vi "stitchingModeOffset.vi"(8 "Offset":dbl, 9 "Data In":dbl[][][](array[numeric])) -> (2 "Stitched Data Out":dbl[][](array[numeric]))   [LabVIEW 2020, in "horiba.lvlib" / "CCD.lvclass"]
doc: "Stitches spectra based on simple cut-off modus."
uses:
  CCD.lvclass
  4c98e68f-fed8-44bd-a6f6-c5aabdf5d44d.vi
  <vilib>/Array/Sort 2D Array - Pop Stack.vi
  <vilib>/Array/Sort 2D Array - Push Stack.vi
  4c98e68f-fed8-44bd-a6f6-c5aabdf5d44d.vi/269d4b3b-47f5-49e3-8884-44851e4dd9d5.vi
  4c98e68f-fed8-44bd-a6f6-c5aabdf5d44d.vi/6d99389c-673d-4efb-bf33-19b32bcf4cf8.vi
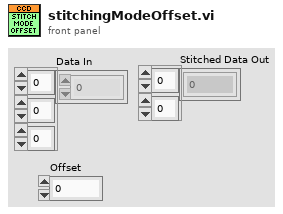
[diagram p1: front panel]
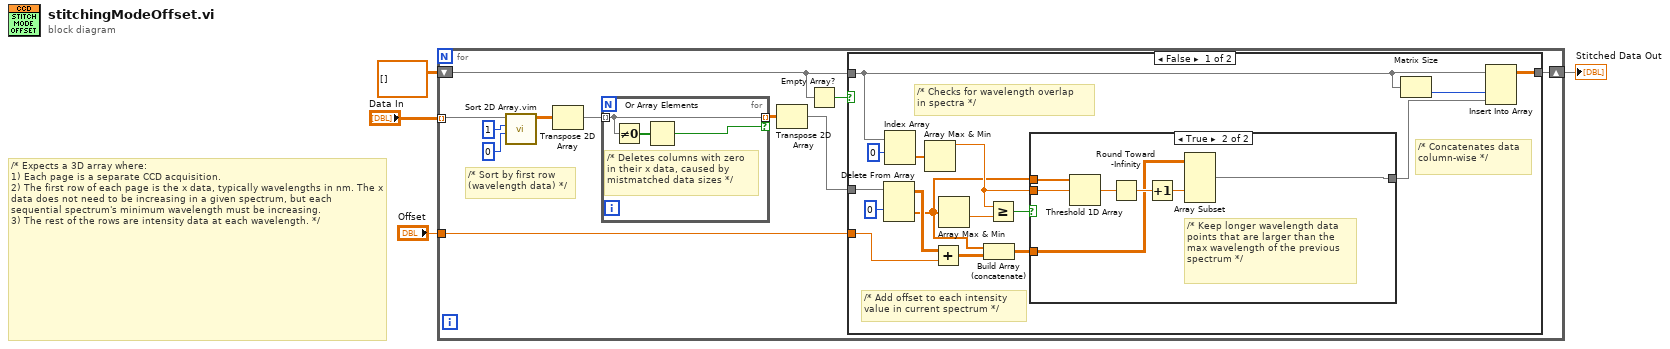
[diagram p0: block diagram]
diagram:
  # "/* Expects a 3D array where:\n1) Each page is a separate CCD acquisition.\n2) The first row of each page is the x data, typically wavelengths in nm. The x data does not need to be increasing in a given spectrum, but each sequential spectrum's minimum wavelength must be increasing.\n3) The rest of the rows are intensity data at each wavelength. */"
  n1 = for {
    tunnel: "Data In" -> [w8] mode=indexing
    shift-right: [w15] -> w4
    shift-left: dbl[][] [] ("Empty Array") -> [w13]
    tunnel: "Offset" -> [w5]
    # "/* Sort by first row \n(wavelength data) */"
    n2 = call "Sort 2D Array.vim"("index"=0, "dimension to index (column)"=1 ("index"), "2D array"=w8) -> ("sorted 2D array"=w7:dbl[][])  [unwired: 7 in, 1 out]
    n3 = Transpose 2D Array(2D array=w7) -> (transposed array=w12:dbl[][])
    n4 = for {
      tunnel: w12 -> [w17] mode=indexing
      tunnel: [w17] -> w11 mode=indexing if=w18
      # "/* Deletes columns with zero\nin their x data, caused by\nmistmatched data sizes */"
      n5 = Not Equal To 0?(x=w17) -> (x != 0?=w16:bool[])
      n6 = Or Array Elements(Boolean array=w16) -> (logical OR=w18:bool)
    }
    n7 = Transpose 2D Array(2D array=w11) -> (transposed array=w6:dbl[][])
    n8 = Empty Array?(array=w13) -> (empty?=w14:bool)
    n9 = case shown="False" w14 {
      tunnel: [w29 w43] -> w15
      tunnel: w6 -> [w26 w43]
      tunnel: w13 -> [w19 _]
      tunnel: w5 -> [w20 _]
      frame False {
        # "/* Add offset to each intensity \nvalue in current spectrum */"
        # "/* Concatenates data \ncolumn-wise */"
        # "/* Checks for wavelength overlap \nin spectra */"
        n10 = Delete From Array(array=w26, index (row)=0) -> (deleted portion=w23:dbl[], array with subset deleted=w24:dbl[][])  [unwired: 2 in]
        n11 = Index Array(array=w19, index (row)=0) -> (element=w32:dbl[])  [unwired: 1 in]
        n12 = Array Max & Min(array=w32) -> (max value=w28:dbl)  [unwired: 3 out]
        n13 = Add(x=w24, y=w20) -> (x+y=w22:dbl[][])
        n14 = Array Max & Min(array=w23) -> (min value=w31:dbl)  [unwired: 3 out]
        n15 = Build Array (concatenate)(w23, w22) -> (w21:dbl[][])
        n16 = Greater Or Equal?(x=w28, y=w31) -> (x >= y?=w30:bool)
        n17 = case shown="True" w30 {
          tunnel: w28 -> [_ w39]
          tunnel: w23 -> [_ w38]
          tunnel: w21 -> [w35 w37]
          tunnel: [w35 w36] -> w27
          frame False {
            # "/* Passes new data unmodified if \nthere is no overlap */"
          }
          frame True {
            # "/* Keep longer wavelength data points that are larger than the max wavelength of the previous spectrum */"
            n18 = Threshold 1D Array(2:w39, 3:w38) -> (0:w41:dbl)  [unwired: 1 in]
            n19 = Round Toward -Infinity(1:w41) -> (0:w42:dbl)
            n20 = Increment(x=w42) -> (x+1=w40:dbl)
            n21 = Array Subset(array=w37, index (col)=w40) -> (w36:dbl[][])  [unwired: 3 in]
          }
        }
        n22 = Matrix Size(0:w19) -> (2:w33:i32)  [unwired: 1 out]
        n23 = Insert Into Array(array=w19, index (col)=w33, new element=w27) -> (w29:dbl[][])  [unwired: 1 in]
      }
      frame True {
        # "/* This case will run on the first loop iteration */"
      }
    }
  }
  "Stitched Data Out" <- w4
